vi "Build Channel Name.vi"(3 "String in":string, 4 "Numeric":i32) -> (9 "String out":string)   [LabVIEW 2014]
doc: "<B>Copyright</B>: (c) MHWirth 2015. All rights reserved.\n\nThis subVI builds a string in the following way: 'String in'_'Numeric'"
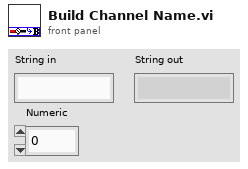
[diagram p1: front panel]
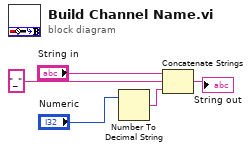
[diagram p0: block diagram]
diagram:
  n1 = Number To Decimal String(number="Numeric") -> (decimal integer string=w5:string)  [unwired: 1 in]
  n2 = Concatenate Strings("String in", "_" ("string"), w5) -> (→"String out":string)
